vi "niRFUtil MASMT 2D Cross Correlation (SGL).vi"(8 "error in (no error)":errorcluster, 9 "algorithm":i32(ring)=1 items=["Direct", "Frequency Domain"], 10 "Y":sgl[][](array[numeric]), 11 "X":sgl[][](array[numeric])) -> (0 "error out":errorcluster, 3 "Rxy":sgl[][](array[numeric]))   [LabVIEW 2015, in "niRFUtil.lvlib"]
doc: "Computes the cross correlation of the input sequences <B>X</B> and <B>Y</B>."
uses:
  niRFUtil.lvlib
  Utilities/niRFMASMT_FFT.dll
panel:
  out "FreqWorkH":sgl[](array[numeric])
  out "WorkH":sgl[](array[numeric])
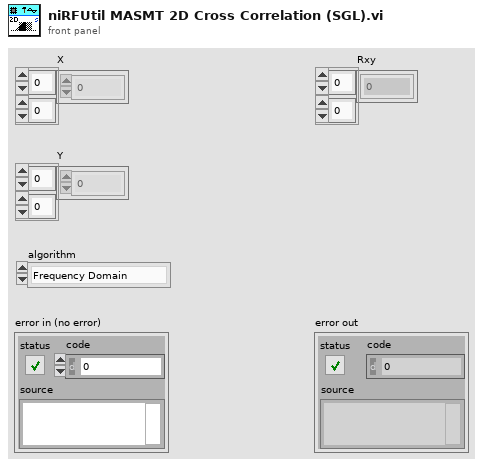
[diagram p1: front panel]
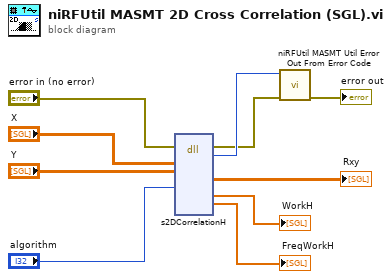
[diagram p0: block diagram]
diagram:
  n1 = dll-call lib="C:/Perforce/semoore-sales/Customers/NATI-3813/Noise Floor/LV Filters/ParallelComplexFilterRFUtil/niRFUtil/MASMT/Utilities/niRFMASMT_FFT.*" fn="s2DCorrelationH"(error in="error in (no error)", "X"="X", "Y"="Y", "domain"="algorithm") -> (error out=w3:errorcluster, "error"=w5:i32, "Rxy"=→"Rxy":sgl[][], "tWorkH"=→"WorkH":sgl[], "tFreqWorkH"=→"FreqWorkH":sgl[])  [unwired: 10 in, 1 out]
  n2 = call "niRFUtil MASMT Util Error Out From Error Code.vi"("error in (no error)"=w3, "error code"=w5) -> ("error out"=→"error out":errorcluster)  [unwired: 9 in]
